vi "AuMT8852B EDR Carrier Frequency and Modulation Results.vi"(8 "error in (no error)":errorcluster, 11 "VISA session":refnum<visa-resource-name>) -> (0 "error out":errorcluster, 2 "error code":i32, 3 "VISA session out":refnum<visa-resource-name>, 4 "Results":T1)   [LabVIEW 2017]
doc: "Anritsu MT8852B Bluetooth Tester\n\nReturns the summary results of the EDR Carrier Frequency Stability and Modulation test.\n\nOUTPUT\nResults - measurements made during the test."
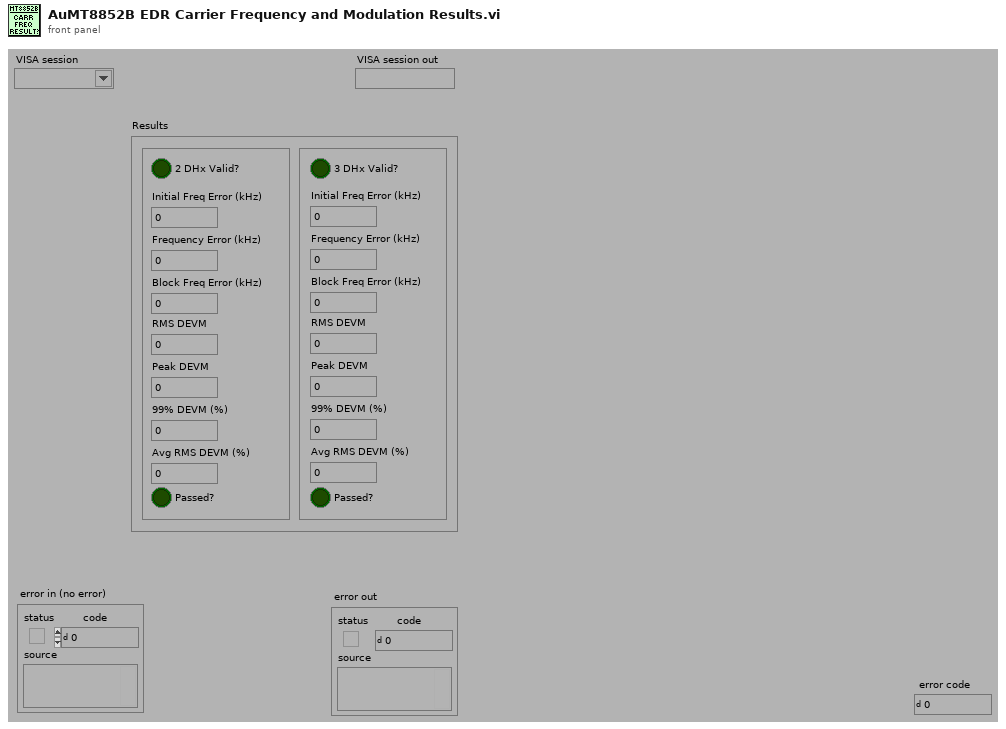
[diagram p1: front panel]
types:
  T1 = cluster{"Passed?":bool, "RMS DEVM":sgl, "Peak DEVM":sgl, "99% DEVM (%)":sgl, "Avg RMS DEVM (%)":sgl, "Initial Freq Error (kHz)":sgl, "Frequency Error (kHz)":sgl, "Block Freq Error (kHz)":sgl, "2 DHx Valid?":bool, "Passed?":bool, "RMS DEVM":sgl, "Peak DEVM":sgl, "99% DEVM (%)":sgl, "Avg RMS DEVM (%)":sgl, "Initial Freq Error (kHz)":sgl, "Frequency Error (kHz)":sgl, "Block Freq Error (kHz)":sgl, "3 DHx Valid?":bool}
  T2 = enum16{"Simulate", "Range check", "Cache", "Query instrument status"}
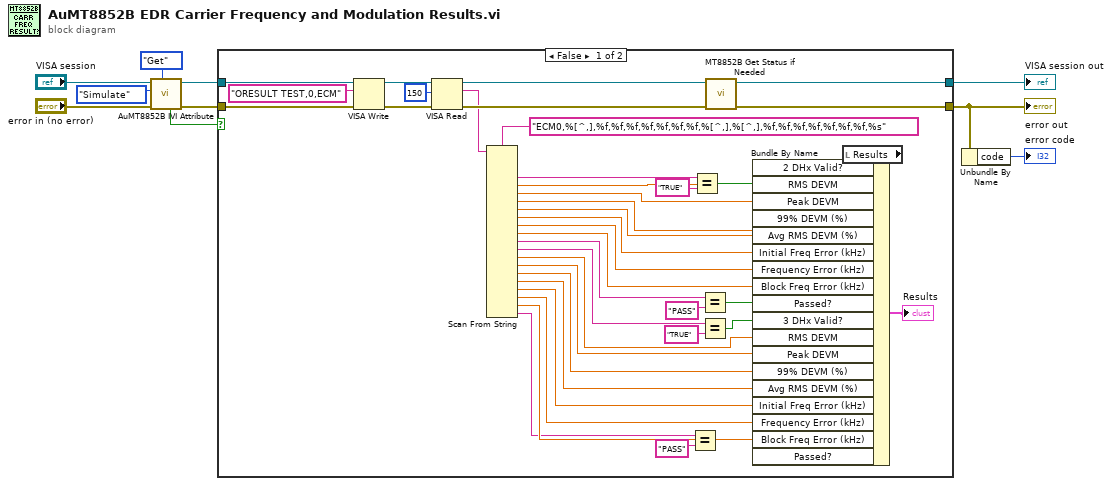
[diagram p0: block diagram]
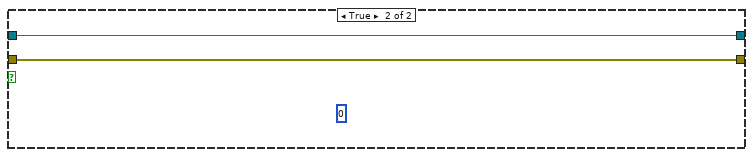
[diagram p2: hidden frame]
diagram:
  n1 = call <instrlib>:"AuMT8852B IVI Attribute.vi"("Set/Get (Set)"=enum16{"Set", "Get"}."Get", "error in (no error)"="error in (no error)", "Flag (Simulate)"=T2."Simulate", "VISA session"="VISA session") -> ("error out"=w7:errorcluster, "VISA session out"=w9:refnum<visa-resource-name>, "Value out"=w3:bool)  [unwired: 5 in]
  n2 = case shown="False" w3 {
    tunnel: [w42 w52] -> w10
    tunnel: [w41 w51] -> w1
    tunnel: w9 -> [w49 w52]
    tunnel: w7 -> [w48 w51]
    frame False {
      n3 = VISA Write(VISA resource name=w49, write buffer="ORESULT TEST,0,ECM" ("write buffer (\"\")"), error in (no error)=w48) -> (VISA resource name out=w47:refnum<visa-resource-name>, error out=w46:errorcluster)  [unwired: 1 out]
      n4 = VISA Read(VISA resource name=w47, byte count=u32 150 ("byte count (0)"), error in (no error)=w46) -> (VISA resource name out=w40:refnum<visa-resource-name>, read buffer=w38:string, error out=w39:errorcluster)  [unwired: 1 out]
      n5 = Scan From String(format string="ECM0,%[^,],%f,%f,%f,%f,%f,%f,%f,%[^,],%[^,],%f,%f,%f,%f,%f,%f,%f,%s" ("Format String"), input string=w38) -> (output 1=w37:string, output 2=w33:dbl, output 3=w32:dbl, output 4=w31:dbl, output 5=w29:dbl, output 6=w28:dbl, output 7=w27:dbl, output 8=w26:dbl, output 9=w25:string, output 10=w20:string, output 11=w19:dbl, output 12=w18:dbl, output 13=w17:dbl, output 14=w16:dbl, output 15=w15:dbl, output 16=w14:dbl, output 17=w13:dbl, output 18=w12:string)  [unwired: 20 in, 3 out]
      n6 = Equal?(x=w12, y="PASS") -> (x = y?=w11:bool)
      n7 = Equal?(x=w37, y="TRUE") -> (x = y?=w34:bool)
      n8 = Equal?(x=w25, y="PASS") -> (x = y?=w23:bool)
      n9 = Equal?(x=w20, y="TRUE") -> (x = y?=w22:bool)
      n10 = call <instrlib>:"MT8852B Get Status if Needed.vi"("error in (no error)"=w39, "VISA session"=w40) -> ("error out"=w41:errorcluster, "VISA session out"=w42:refnum<visa-resource-name>)  [unwired: 8 in]
      n11 = local read "Results"() -> (w35:T1)
      n12 = Bundle By Name(cluster=w35, "2 DHx Valid?"=w34, "RMS DEVM"=w33, "Peak DEVM"=w32, "99% DEVM (%)"=w31, "Avg RMS DEVM (%)"=w29, "Initial Freq Error (kHz)"=w28, "Frequency Error (kHz)"=w27, "Block Freq Error (kHz)"=w26, "Passed?"=w23, "3 DHx Valid?"=w22, "RMS DEVM"=w19, "Peak DEVM"=w18, "99% DEVM (%)"=w17, "Avg RMS DEVM (%)"=w16, "Initial Freq Error (kHz)"=w15, "Frequency Error (kHz)"=w14, "Block Freq Error (kHz)"=w13, "Passed?"=w11) -> (→"Results":T1)
    }
    frame True {
      (unwired) u8 0
    }
  }
  "error out" <- w1
  "VISA session out" <- w10
  n13 = Unbundle By Name(w1) -> ("code"=→"error code":i32)
